vi "Global 1.vi"() -> ()   [LabVIEW 2014]
panel:
  in  "Stacker 2 Encoder Change":dbl
  in  "Auto Claw":bool
  in  "Min Elevator Value":dbl
  in  "Lock T":bool
  in  "Negative Reset":dbl
  in  "Low Level":bool
  in  "High Level":bool
  in  "Manual Elevator":dbl
  in  "Manual Mode":bool
  in  "Switch Mode":bool
  in  "Elevator Down":bool
  in  "Switch Speed":bool
  in  "Half Speed":bool
  in  "Flying T Axis":dbl
  in  "Flying T Piston":bool
  in  "Test Flying T":bool
  in  "Elevator Up":bool
  in  "Open/Close T":bool
  in  "Pot Volt":dbl
  in  "Fudge Encoder Value":dbl
  in  "Piston 2":bool
  in  "Piston 1":bool
  in  "Grab Both":bool
  in  "Total Encoder Value":dbl
  in  "Payload Encoder Value":dbl
  in  "Target Encoder Value":dbl
  in  "Setpoint Encoder Value":dbl
  in  "Payload Number":dbl
  in  "Target Number":dbl
  in  "Setpoint Level":dbl
  in  "Cycle Payload":bool
  in  "Cycle Target":bool
  in  "Fudge":dbl
  in  "Level Down":bool
  in  "Level Up":bool
  in  "Auto-Stack":bool
  in  "Speed Right":dbl
  in  "Speed Left":dbl
  in  "X-Axis Joystick 1":dbl
  in  "X-Axis Joystick 0":dbl
  in  "Outake":bool
  in  "Intake":bool
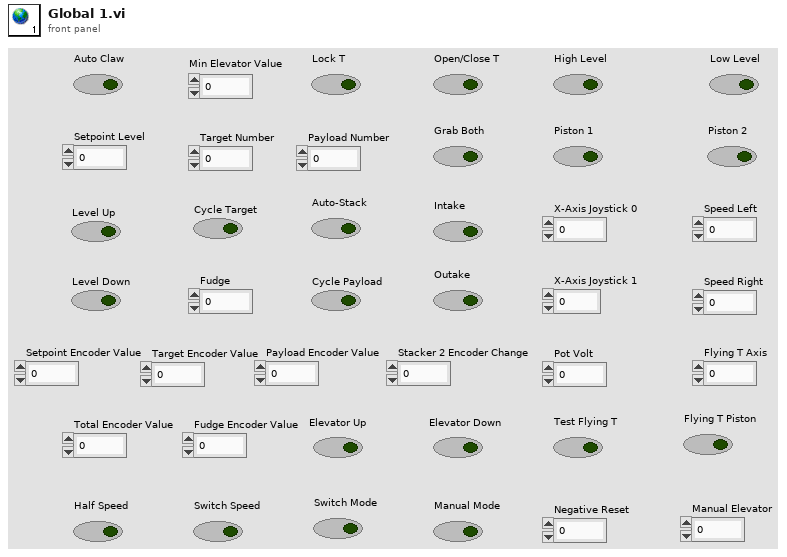
[diagram p1: front panel]
diagram:
